vi "Get Clients.vi"(8 "error in (no error)":errorcluster, 11 "Chat Server in":refnum<class "Chat Server.lvclass">) -> (0 "error out":errorcluster, 2 "Connections":refnum<class "Connection.lvclass">[](array[class]), 3 "Chat Server out":refnum<class "Chat Server.lvclass">)   [LabVIEW 2020, in "Chat Server.lvclass"]
uses:
  Chat Server.lvclass
  lv-stream/stream/Connection/Connection.lvclass
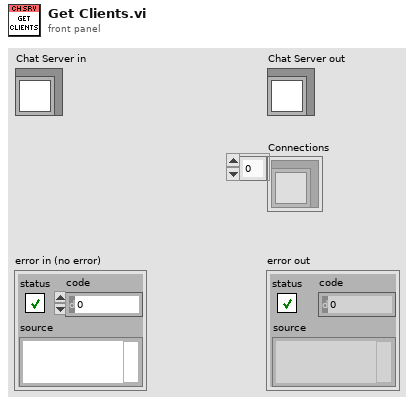
[diagram p1: front panel]
types:
  T1 = typedef "Chat Server.lvclass/Red Data.ctl" = cluster{"Connections":refnum<class "Connection.lvclass">[]}
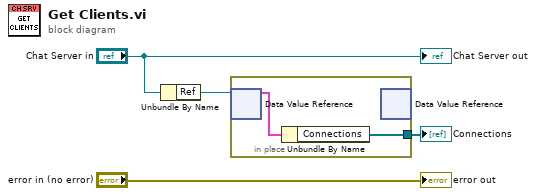
[diagram p0: block diagram]
diagram:
  n1 = Unbundle By Name("Chat Server in") -> ("Ref"=w3:refnum<data-value>)
  n2 = in-place {
    in-place-border: [w5] -> w1
    n3 = in-place-dvr #1(w3) -> (w6:T1)  [unwired: 1 out]
    n4 = Unbundle By Name(w6) -> ("Connections"=w5:refnum<class "Connection.lvclass">[])
    n5 = in-place-dvr #1() -> ()  [unwired: 1 in, 2 out]
  }
  "Connections" <- w1
  "error out" <- "error in (no error)"
  "Chat Server out" <- "Chat Server in"
